vi "UIStep Configure UI.vi"(8 "error in (no error)":errorcluster, 10 "Project In":refnum<class "Project.lvclass">, 11 "SerializableObject in":refnum<class>) -> (0 "error out":errorcluster, 3 "SerializableObject out":refnum<class>)   [LabVIEW 2015, in "UIStep.lvclass"]
uses:
  UIStep.lvclass
  Project.lvclass
  SerializableObject/CONFIGURE_UI_STATE.ctl
  Step.lvclass
  Editor/Editor.lvclass
panel:
  in  "Name":string
  in  "Stop If Fail":bool
  in  "Skip":bool
  in  "OutputPanelBtn":bool
  in  "UISettingPanelBtn":bool
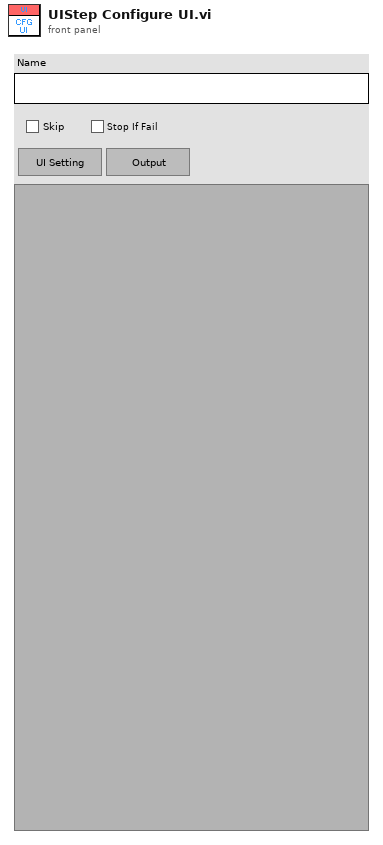
[diagram p1: front panel]
types:
  T1 = typedef "Editor.lvclass/CONFIGURE_UI_STATE.ctl" = enum16{"UI_LOOP", "INIT", "END", "CHANGE_PANEL"}
  T2 = enum8{"Enabled", "Disabled", "Disabled and Grayed Out"}
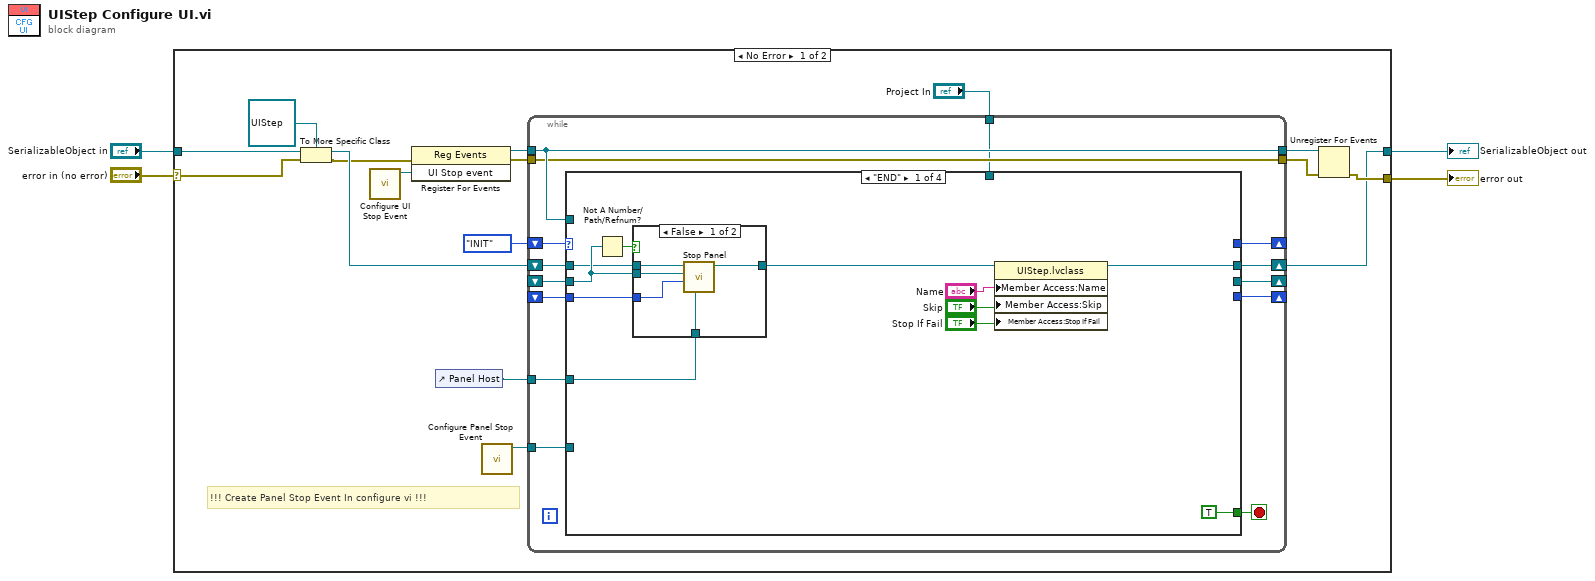
[diagram p0: block diagram]
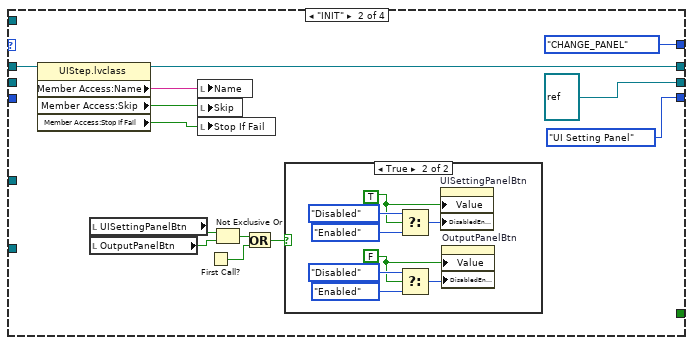
[diagram p3: hidden frame]
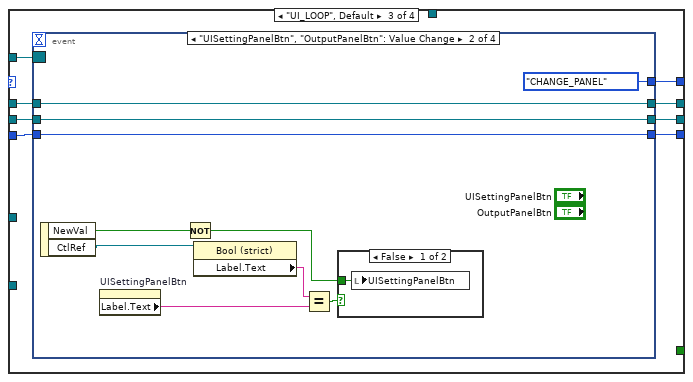
[diagram p5: hidden frame]
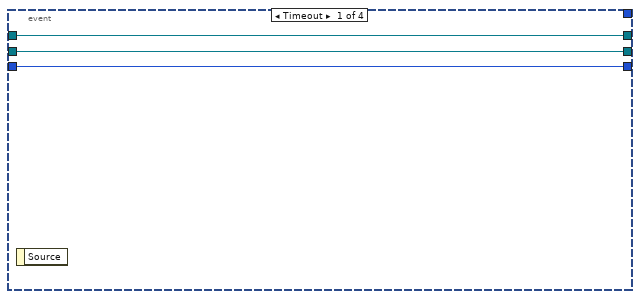
[diagram p6: hidden frame]
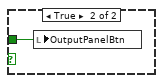
[diagram p7: hidden frame]
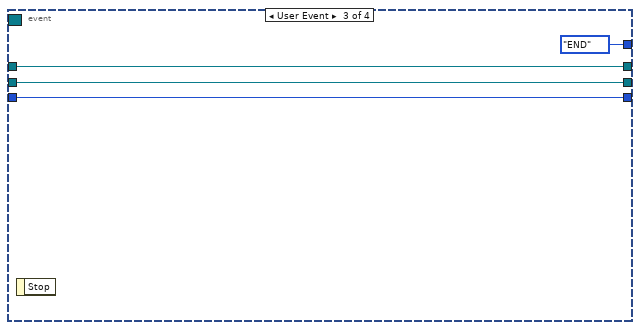
[diagram p8: hidden frame]
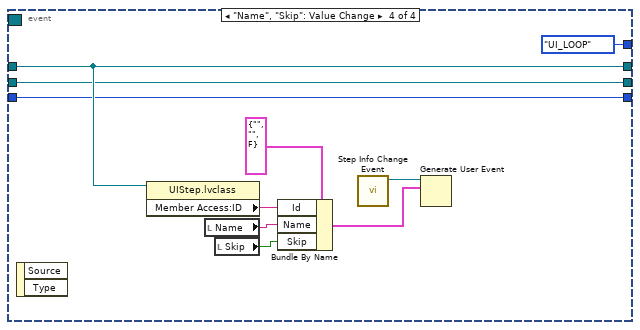
[diagram p9: hidden frame]
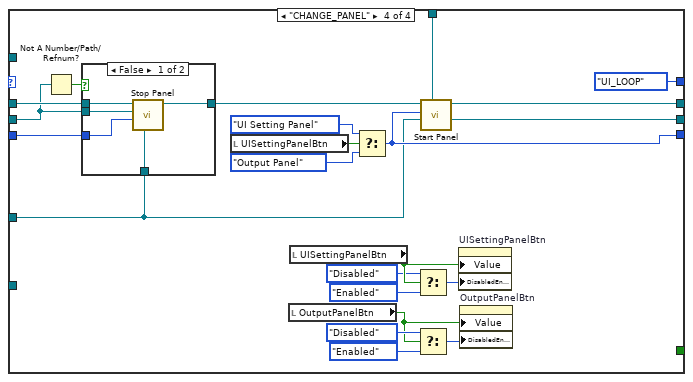
[diagram p10: hidden frame]
diagram:
  n1 = case shown="No Error" "error in (no error)" {
    selector: "error in (no error)" -> [w18 w139]
    tunnel: [w12 w139] -> w3
    tunnel: "SerializableObject in" -> [w20 w138]
    tunnel: [w11 w138] -> w1
    frame No Error {
      # "!!! Create Panel Stop Event In configure vi !!!"
      n2 = To More Specific Class(target class=refnum<class "UIStep.lvclass"> refnum ("ConfigureableObject in"), reference=w20, error in=w18) -> (specific class reference=w10:refnum<class "UIStep.lvclass">, error out=w8:errorcluster)
      n3 = call "Configure UI Stop Event.vi"() -> ("UI Stop event"=w9:refnum<user-event>)  [unwired: 11 in]
      n4 = register-events(error in=w8, w9) -> (reference out=w13:refnum<event-registration>, error out=w15:errorcluster)  [unwired: 1 in]
      n5 = control-ref of="Panel Host"() -> (w5:refnum<vi>)
      n6 = call "Configure Panel Stop Event.vi"() -> ("Panel Stop event"=w7:refnum<user-event>)  [unwired: 11 in]
      n7 = while {
        tunnel: w13 -> [w34]
        tunnel: [w34] -> w14
        tunnel: w15 -> [w33]
        tunnel: [w33] -> w16
        shift-right: [w31] -> w11
        shift-left: w10 -> [w32]
        shift-right: [w29] -> _
        shift-left: CONFIGURE_UI_STATE."INIT" -> [w30]
        tunnel: w7 -> [w27]
        shift-right: [w26] -> _
        shift-left: _ -> [w23]
        shift-right: [w25] -> _
        shift-left: _ -> [w24]
        tunnel: "Project In" -> [w22]
        tunnel: w5 -> [w21]
        stop <- w28 stop-if-true
        n8 = case shown="\"END\"" w30 {
          tunnel: w34 -> [_ _ w80 _]
          tunnel: w32 -> [w37 w64 w79 w121]
          tunnel: [w44 w63 w78 w116] -> w31
          tunnel: [_ CONFIGURE_UI_STATE."CHANGE_PANEL" w77 CONFIGURE_UI_STATE."UI_LOOP"] -> w29
          tunnel: [TRUE _ _ _] -> w28
          tunnel: w27 -> [_ _ _ _]
          tunnel: [_ enum16{"UI Setting Panel", "Output Panel"}."UI Setting Panel" ("Panel") w76 w111] -> w26
          tunnel: [_ refnum<vi> refnum ("Panel VI out") w73 w115] -> w25
          tunnel: w24 -> [w39 _ w74 w120]
          tunnel: w23 -> [w38 _ w75 w119]
          tunnel: w22 -> [_ _ _ w117]
          tunnel: w21 -> [w35 _ _ w110]
          frame "END" {
            n9 = Not A Number/Path/Refnum?(number/path/refnum=w39) -> (NaN/Path/Refnum?=w40:bool)
            n10 = case shown="False" w40 {
              tunnel: w37 -> [w50 w51]
              tunnel: w39 -> [w49 _]
              tunnel: w38 -> [w48 _]
              tunnel: w35 -> [w47 _]
              tunnel: [w46 w51] -> w36
              frame False {
                n11 = call "Stop Panel.vi"("Panel Host"=w47, "Panel"=w48, "Panel VI in"=w49, "UIStep in"=w50) -> ("UIStep out"=w46:refnum<class "UIStep.lvclass">)  [unwired: 6 in, 1 out]
              }
              frame True {
              }
            }
            n12 = property class="UIStep.lvclass"(reference=w36, "Member Access:Name"="Name", "Member Access:Skip"="Skip", "Member Access:Stop If Fail"="Stop If Fail") -> (reference out=w44:refnum<class "UIStep.lvclass">)  [unwired: 1 in, 1 out]
          }
          frame "INIT" {
            n13 = property class="UIStep.lvclass"(reference=w64) -> (reference out=w63:refnum<class "UIStep.lvclass">, "Member Access:Name"=w62:string, "Member Access:Skip"=w61:bool, "Member Access:Stop If Fail"=w60:bool)  [unwired: 1 in, 1 out]
            n14 = local read "UISettingPanelBtn"() -> (w55:bool)
            n15 = local read "OutputPanelBtn"() -> (w54:bool)
            n16 = local write "Name"(w62) -> ()
            n17 = local write "Skip"(w61) -> ()
            n18 = local write "Stop If Fail"(w60) -> ()
            n19 = First Call?() -> (First Call?: T/F=w57:bool)
            n20 = Not Exclusive Or(1:w54, 2:w55) -> (0:w56:bool)
            n21 = Or(x=w56, y=w57) -> (x .or. y?=w58:bool)
            n22 = case shown="True" w58 {
              frame False {
              }
              frame True {
                w65 = FALSE
                w66 = TRUE
                n23 = Select(t=T2."Disabled" ("Disabled"), s=w66, f=T2."Enabled" ("Disabled")) -> (s? t:f=w71:T2)
                n24 = Select(t=T2."Disabled" ("Disabled"), s=w65, f=T2."Enabled" ("Disabled")) -> (s? t:f=w67:T2)
                n25 = property on="UISettingPanelBtn" class="Bool (strict)"("Value"=w66, "DisabledEnum"=w71) -> ()  [unwired: 2 in, 2 out]
                n26 = property on="OutputPanelBtn" class="Bool (strict)"("Value"=w65, "DisabledEnum"=w67) -> ()  [unwired: 2 in, 2 out]
              }
            }
          }
          frame "UI_LOOP", Default {
            n27 = event shown="[1] \"UISettingPanelBtn\", \"OutputPanelBtn\": Value Change" {
              selector: w80 -> [_ _ _ _]
              dyn-events: _ -> [_ _ _ _]
              timeout: _ -> [_ _ _ _]
              tunnel: w79 -> [w83 w93 w99 w104]
              tunnel: [w83 w93 w99 w104] -> w78
              tunnel: [_ CONFIGURE_UI_STATE."CHANGE_PANEL" CONFIGURE_UI_STATE."END" CONFIGURE_UI_STATE."UI_LOOP"] -> w77
              tunnel: [w82 w85 w97 w101] -> w76
              tunnel: w75 -> [w82 w85 w97 w101]
              tunnel: [w81 w84 w96 w100] -> w73
              tunnel: w74 -> [w81 w84 w96 w100]
              event Timeout {
                n28 = event-data() -> ()  [unwired: 1 in, 1 out]
              }
              event "UISettingPanelBtn", "OutputPanelBtn": Value Change {
                n29 = event-data() -> ("NewVal"=w87:bool, "CtlRef"=w86:refnum<vi>)  [unwired: 1 in]
                n30 = property on="UISettingPanelBtn" class="Bool (strict)"() -> ("Label.Text"=w88:string)  [unwired: 2 in, 2 out]
                n31 = Not(x=w87) -> (.not. x?=w89:bool)
                n32 = property class="Bool (strict)"(reference=w86) -> ("Label.Text"=w91:string)  [unwired: 1 in, 2 out]
                n33 = Equal?(x=w91, y=w88) -> (x = y?=w90:bool)
                n34 = case shown="False" w90 {
                  tunnel: w89 -> [w94 w95]
                  frame False {
                    n35 = local write "UISettingPanelBtn"(w94) -> ()
                  }
                  frame True {
                    n36 = local write "OutputPanelBtn"(w95) -> ()
                  }
                }
              }
              event User Event {
                n37 = event-data() -> ()  [unwired: 1 in, 1 out]
              }
              event "Name", "Skip": Value Change {
                n38 = event-data() -> ()  [unwired: 1 in, 2 out]
                n39 = property class="UIStep.lvclass"(reference=w104) -> ("Member Access:ID"=w107:string)  [unwired: 1 in, 2 out]
                n40 = local read "Name"() -> (w103:string)
                n41 = local read "Skip"() -> (w102:bool)
                n42 = Bundle By Name(cluster=cluster{"Id":string, "Name":string, "Skip":bool} {"Id"="", "Name"="", "Skip"=FALSE} ("Step Info"), "Id"=w107, "Name"=w103, "Skip"=w102) -> (w105:cluster{"Id":string, "Name":string, "Skip":bool})
                n43 = call "Step Info Change Event.vi"() -> ("Step Info Change Event"=w108:refnum<user-event>)  [unwired: 11 in]
                n44 = Generate User Event(user event=w108, event data cluster=w105) -> ()  [unwired: 2 in, 2 out]
              }
            }
          }
          frame "CHANGE_PANEL" {
            n45 = Not A Number/Path/Refnum?(number/path/refnum=w120) -> (NaN/Path/Refnum?=w122:bool)
            n46 = case shown="False" w122 {
              tunnel: w121 -> [w136 w137]
              tunnel: w120 -> [w135 _]
              tunnel: w119 -> [w134 _]
              tunnel: w110 -> [w133 _]
              tunnel: [w132 w137] -> w118
              frame False {
                n47 = call "Stop Panel.vi"("Panel Host"=w133, "Panel"=w134, "Panel VI in"=w135, "UIStep in"=w136) -> ("UIStep out"=w132:refnum<class "UIStep.lvclass">)  [unwired: 6 in, 1 out]
              }
              frame True {
              }
            }
            n48 = local read "UISettingPanelBtn"() -> (w114:bool)
            n49 = local read "OutputPanelBtn"() -> (w123:bool)
            n50 = local read "UISettingPanelBtn"() -> (w128:bool)
            n51 = Select(t=enum16{"UI Setting Panel", "Output Panel"}."UI Setting Panel" ("Panel"), s=w114, f=enum16{"UI Setting Panel", "Output Panel"}."Output Panel" ("Panel")) -> (s? t:f=w111:enum16{"UI Setting Panel", "Output Panel"})
            n52 = Select(t=T2."Disabled" ("Disabled"), s=w128, f=T2."Enabled" ("Disabled")) -> (s? t:f=w129:T2)
            n53 = Select(t=T2."Disabled" ("Disabled"), s=w123, f=T2."Enabled" ("Disabled")) -> (s? t:f=w124:T2)
            n54 = call "Start Panel.vi"("Project In"=w117, "Panel Host"=w110, "Panel"=w111, "UIStep in"=w118) -> ("Panel VI out"=w115:refnum<vi>, "UIStep out"=w116:refnum<class "UIStep.lvclass">)  [unwired: 5 in, 1 out]
            n55 = property on="UISettingPanelBtn" class="Bool (strict)"("Value"=w128, "DisabledEnum"=w129) -> ()  [unwired: 2 in, 2 out]
            n56 = property on="OutputPanelBtn" class="Bool (strict)"("Value"=w123, "DisabledEnum"=w124) -> ()  [unwired: 2 in, 2 out]
          }
        }
      }
      n57 = Unregister For Events(event registration refnum=w14, error in=w16) -> (error out=w12:errorcluster)
    }
    frame Error {
    }
  }
  "error out" <- w3
  "SerializableObject out" <- w1
